vi "Write Cylinder.vi"(10 "IActuatorCylinder.lvclass":refnum<class "IActuatorCylinder.lvclass">, 11 "PressureServoCylinderActuator in":refnum<class "PressureServoCylinderActuator.lvclass">) -> (3 "PressureServoCylinderActuator out":refnum<class "PressureServoCylinderActuator.lvclass">)   [LabVIEW 2015, in "PressureServoCylinderActuator.lvclass"]
uses:
  PressureServoCylinderActuator.lvclass
  IActuatorCylinder/IActuatorCylinder.lvclass
  PressureServoCylinderActuator.lvclass/PressureServoCylinderActuator.ctl
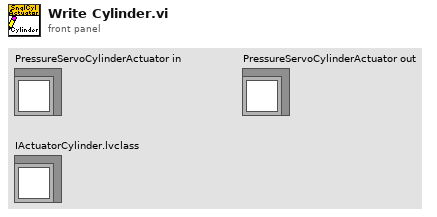
[diagram p1: front panel]
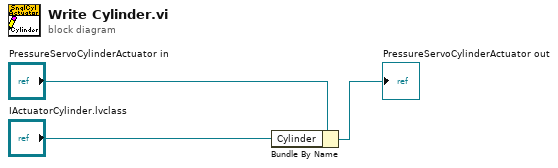
[diagram p0: block diagram]
diagram:
  n1 = Bundle By Name(cluster="PressureServoCylinderActuator in", "Cylinder"="IActuatorCylinder.lvclass") -> (→"PressureServoCylinderActuator out":refnum<class "PressureServoCylinderActuator.lvclass">)
